vi "Get force data.vi"(8 "error in (no error)":errorcluster) -> (0 "error out":errorcluster, 3 "FS Data":dbl)   [LabVIEW 2020]
uses:
  Controls/HW States.ctl
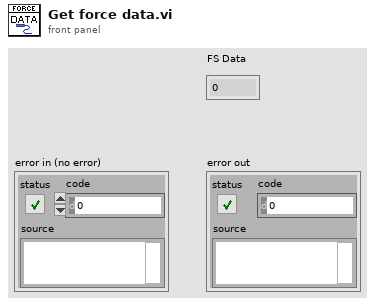
[diagram p1: front panel]
types:
  T1 = typedef "HW States.ctl" = enum16{"Initialize", "Input LED", "Input PWM", "Acquire Voltage", "Acquire Image", "Stop"}
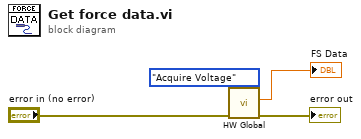
[diagram p0: block diagram]
diagram:
  n1 = call "HW Global.vi"("HW State"=HW_States."Acquire Voltage", "error in (no error)"="error in (no error)") -> ("error out"=→"error out":errorcluster, "FS Data"=→"FS Data":dbl)  [unwired: 6 in, 2 out]
